vi "Test_Save_Image.vi"() -> ()   [LabVIEW 2017]
uses:
  <vilib>/userdefined/High Color/IMAQdx.ctl
panel:
  out "error out":errorcluster
  in  "Session In":T1
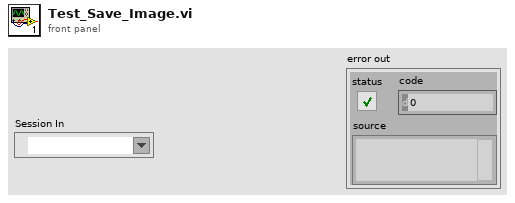
[diagram p1: front panel]
types:
  T1 = typedef "IMAQdx.ctl" = refnum<k21>
  T2 = typedef "IMAQ Image.ctl" = refnum<image>
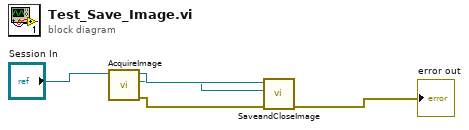
[diagram p0: block diagram]
diagram:
  n1 = call "AcquireImage.vi"("Session In"="Session In") -> ("error out"=w4:errorcluster, "Session Out"=w2:T1, "Image"=w3:T2)  [unwired: 8 in]
  n2 = call "SaveandCloseImage.vi"("error in"=w4, "Session In"=w2, "Image In"=w3) -> ("error out"=→"error out":errorcluster)  [unwired: 8 in]
